vi "GET_issue.vi"(8 "error in (no error)":errorcluster, 10 "issueID":i32, 11 "MyComics.org_class in":refnum<class "MyComics.org_class.lvclass">) -> (0 "error out":errorcluster, 3 "MyComics.org_class out":refnum<class "MyComics.org_class.lvclass">)   [LabVIEW 2024, in "MyComics.org_class.lvclass"]
uses:
  MyComics.org_class.lvclass
  MyComics.org_class.lvclass/MyComics.org_class.ctl
  <vilib>/httpClient/LabVIEWHTTPClient.lvlib
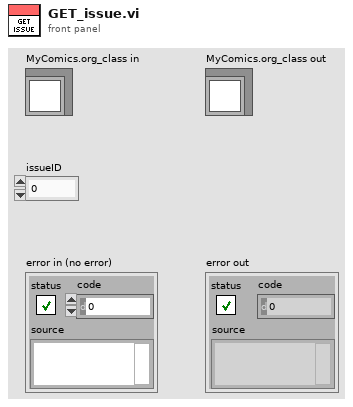
[diagram p1: front panel]
types:
  T1 = typedef "LabVIEWHTTPClient.lvlib/ClientHandle.ctl" = refnum<k1>
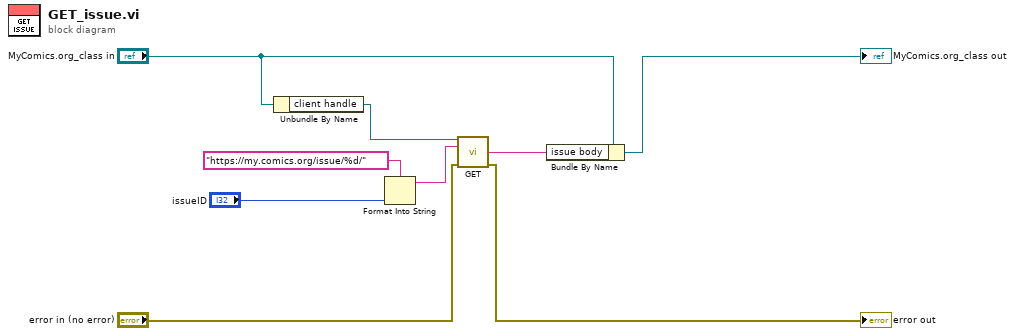
[diagram p0: block diagram]
diagram:
  n1 = Unbundle By Name("MyComics.org_class in") -> ("client handle"=w9:T1)
  n2 = Format Into String(format string="https://my.comics.org/issue/%d/", "issueID") -> (resulting string=w4:string)  [unwired: 2 in, 1 out]
  n3 = call <vilib>:"GET.vi"("client handle"=w9, "url"=w4, "error in (no error)"="error in (no error)") -> ("body"=w1:string, "error out"=→"error out":errorcluster)  [unwired: 9 in, 2 out]
  n4 = Bundle By Name(cluster="MyComics.org_class in", "issue body"=w1) -> (→"MyComics.org_class out":refnum<class "MyComics.org_class.lvclass">)
